vi "Main.vi"() -> ()   [LabVIEW 2019]
uses:
  <vilib>/vision/Image Controls.llb/IMAQ Image.ctl
  <vilib>/vision/NI_Vision_Development_Module.lvlib
panel:
  in  "Save Button":bool
  in  "Clear Button":bool
  in  "Image Path":path=path "D:/Krystian/Krystian/LabVIEW Data/OSP Projekt/Data/1.jpg" caption="Picture Path"
  in  "Exit":bool
  in  "Start":bool
  out "Results":string
  out "Image":T1(plugin-control)
  # "Application Panel"
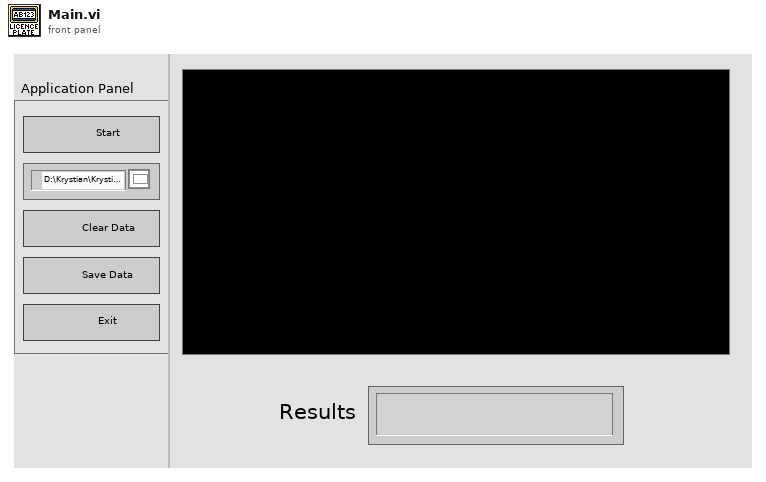
[diagram p1: front panel]
types:
  T1 = typedef "IMAQ Image.ctl" = refnum<image>
  T2 = enum32{"Invalid", "Standard", "Closed", "Hidden", "Minimized", "Maximized"}
  T3 = enum32{"invalid app kind", "Development System", "Run Time System", "Student Edition", "Embedded LabVIEW", "Evaluation", "Custom"}
  T4 = cluster{"Core":cluster{"Current VI Reference":refnum<vi>, "Close Panel on Exit?":bool}, "Your Boolean data":bool, "Results":string, "Image Path":path, "Data":cluster{"Rectangle":i32[]}, "Image":refnum<image>, "Python Path":path}
  T5 = cluster{"Current VI Reference":refnum<vi>, "Close Panel on Exit?":bool}
  T6 = typedef "Image Type" = u32
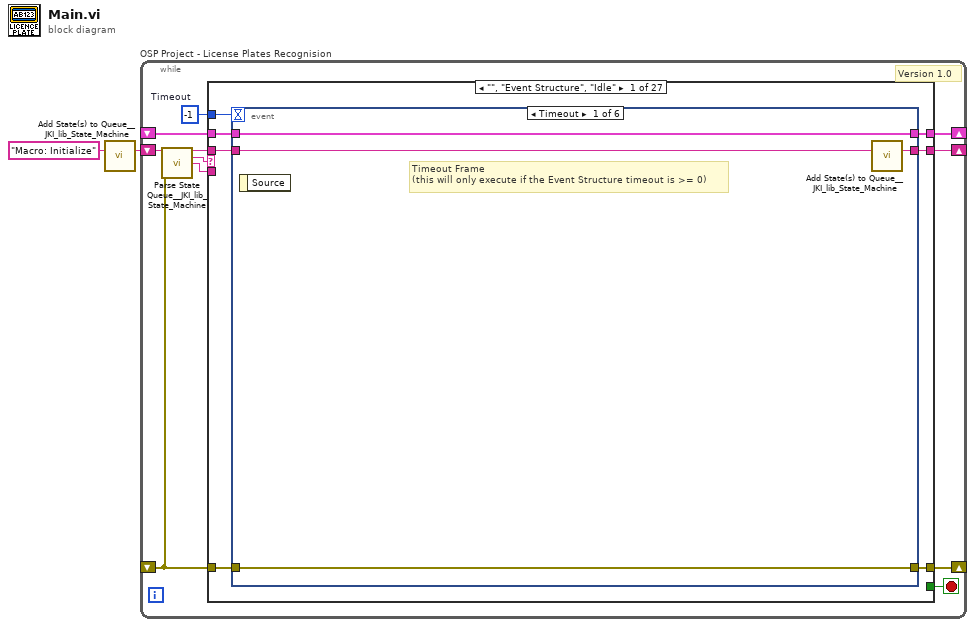
[diagram p0: block diagram]
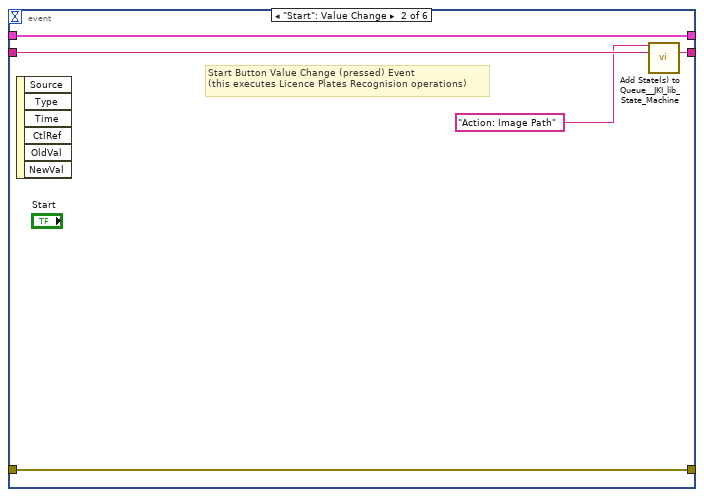
[diagram p2: hidden frame]
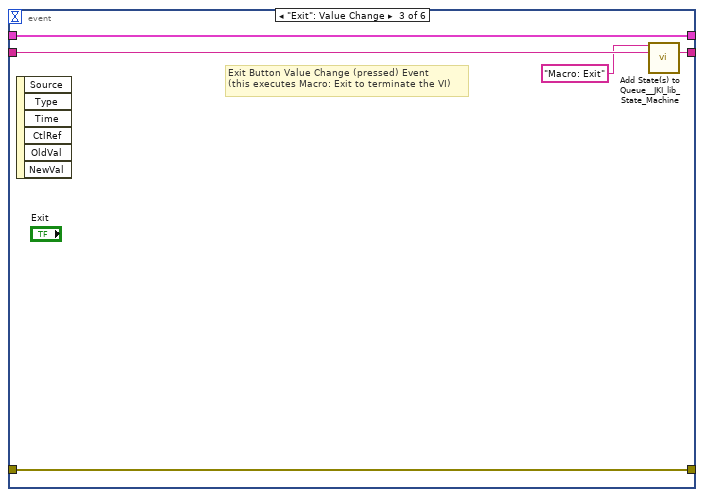
[diagram p3: hidden frame]
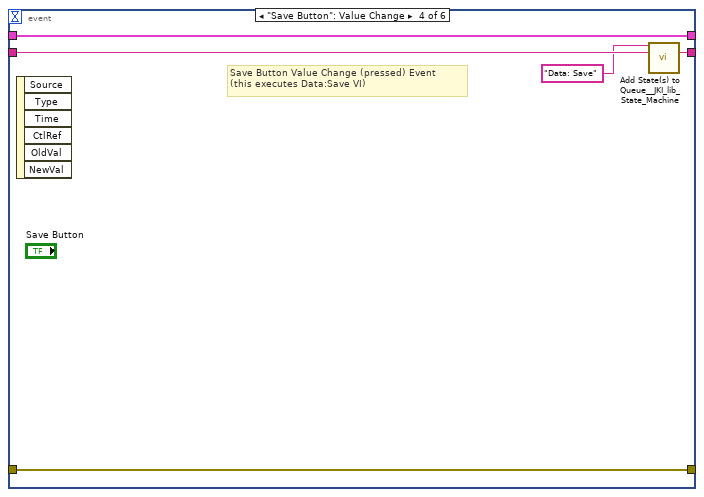
[diagram p4: hidden frame]
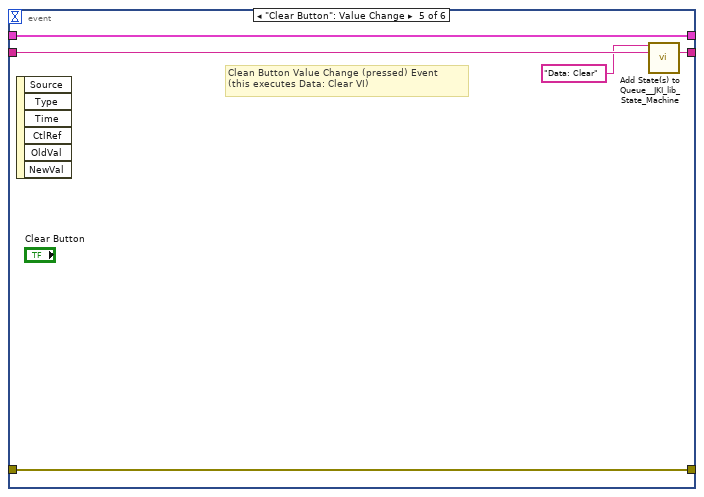
[diagram p5: hidden frame]
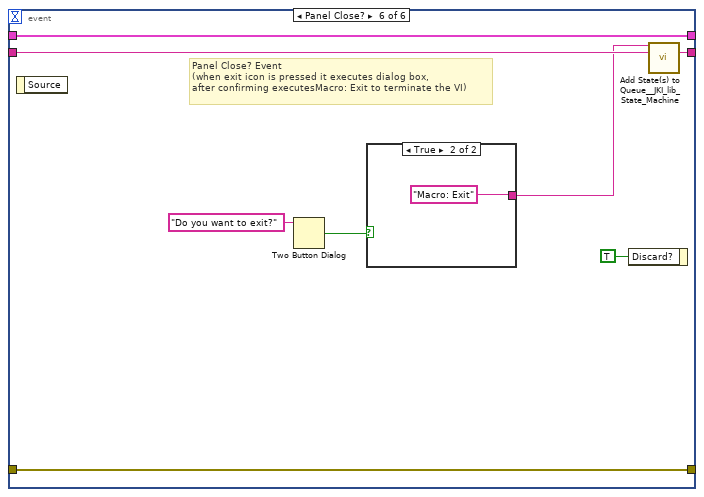
[diagram p6: hidden frame]
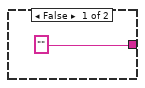
[diagram p7: hidden frame]
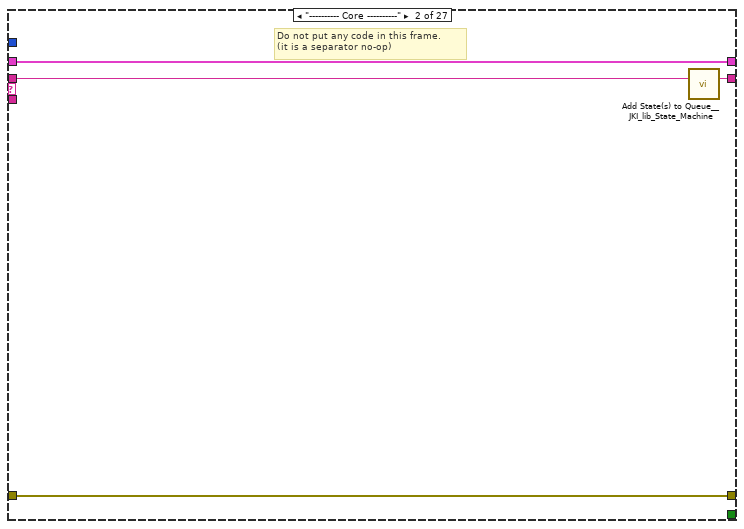
[diagram p8: hidden frame]
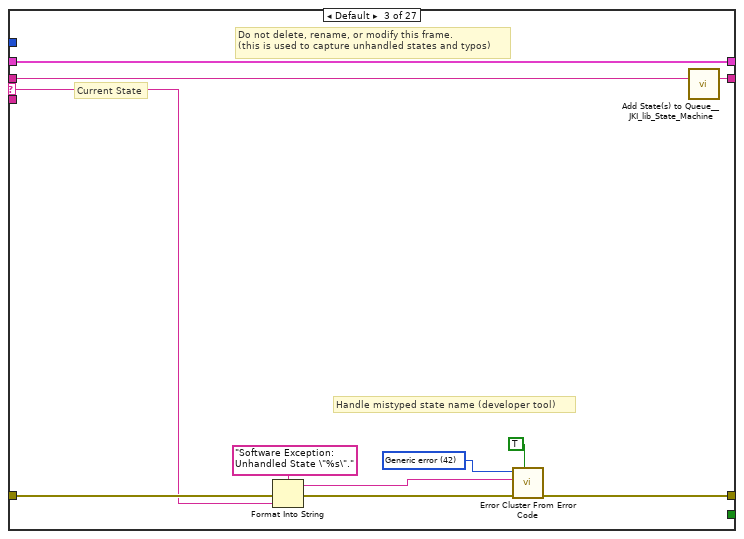
[diagram p9: hidden frame]
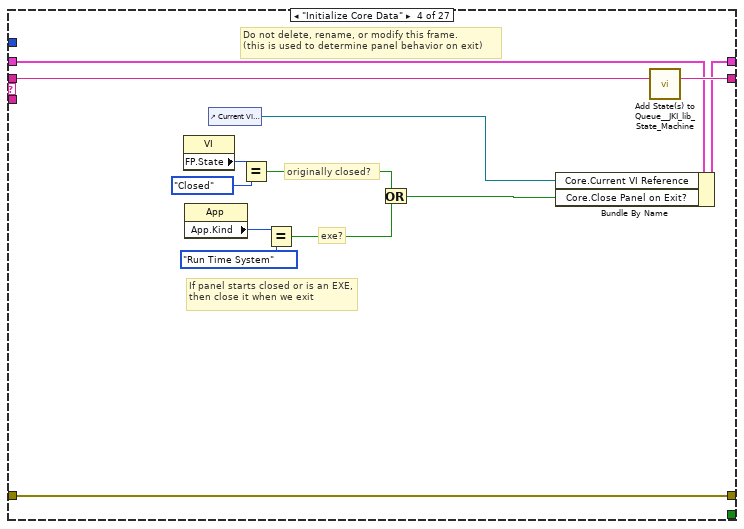
[diagram p10: hidden frame]
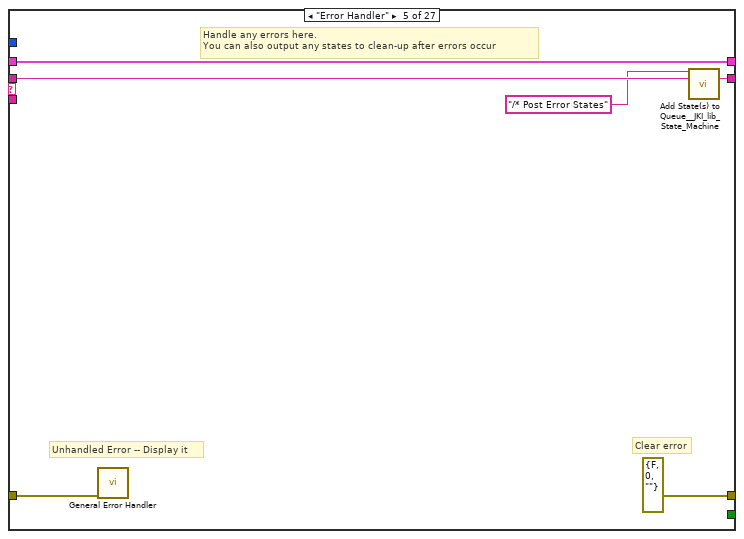
[diagram p11: hidden frame]
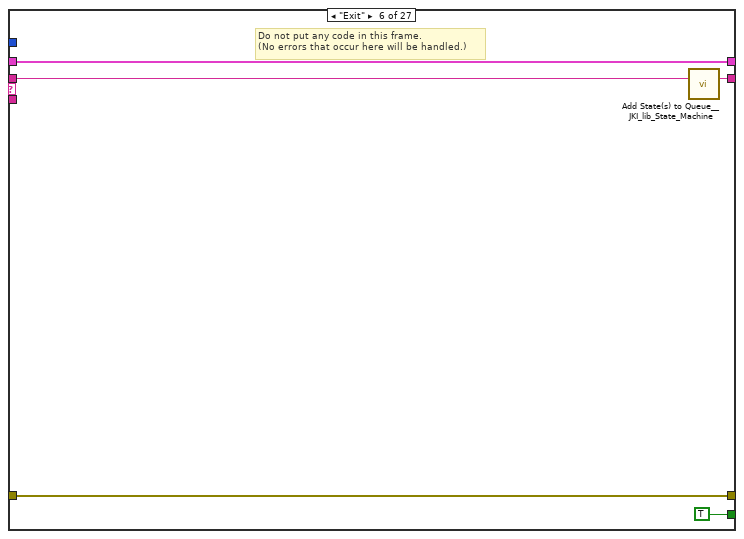
[diagram p12: hidden frame]
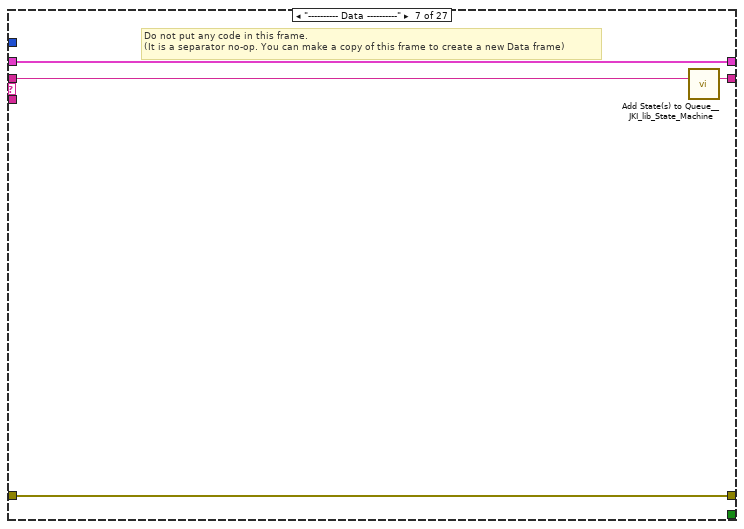
[diagram p13: hidden frame]
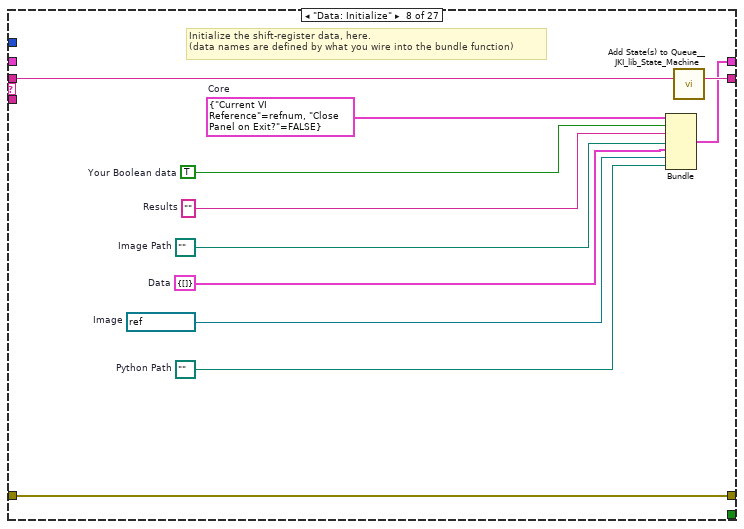
[diagram p14: hidden frame]
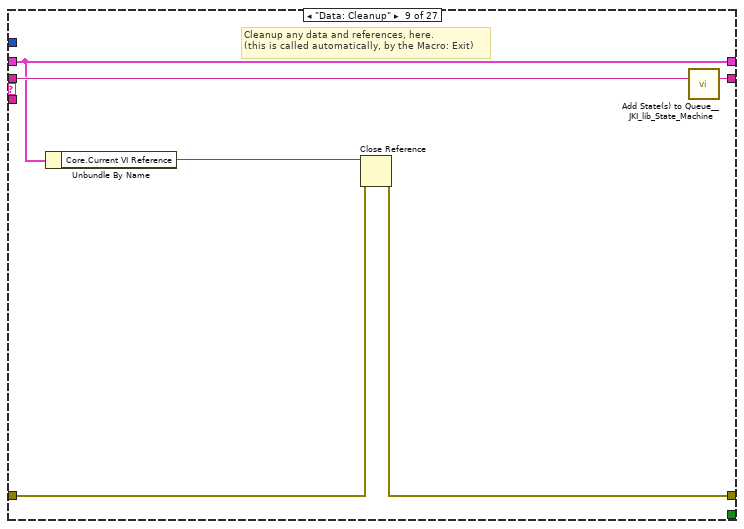
[diagram p15: hidden frame]
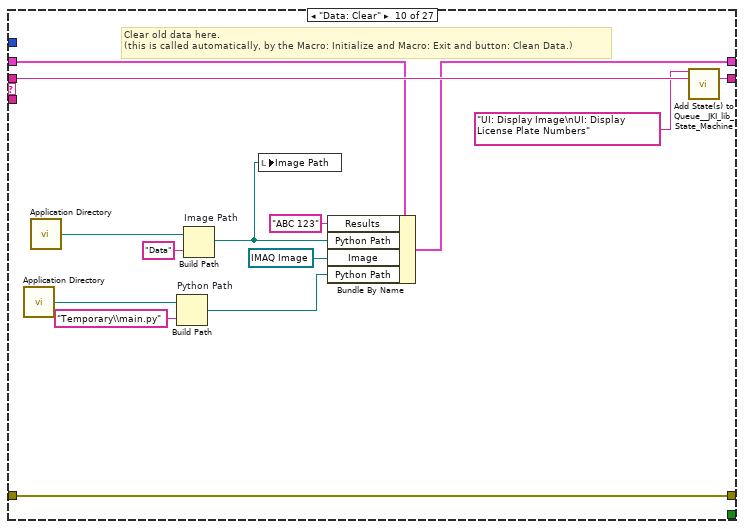
[diagram p16: hidden frame]
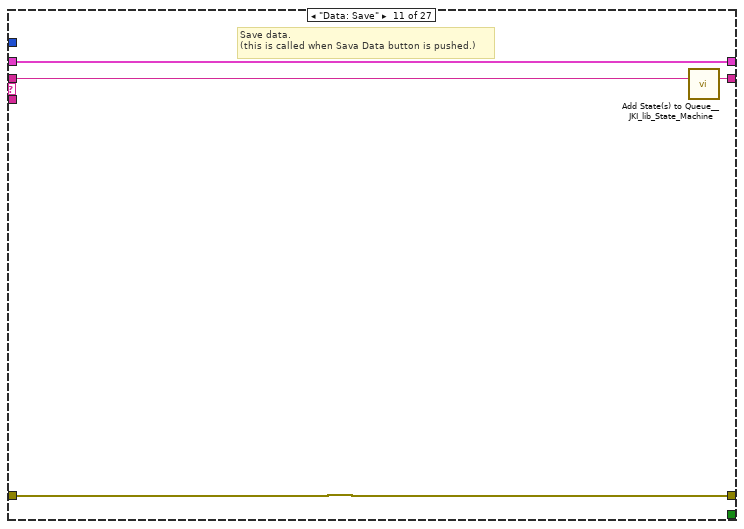
[diagram p17: hidden frame]
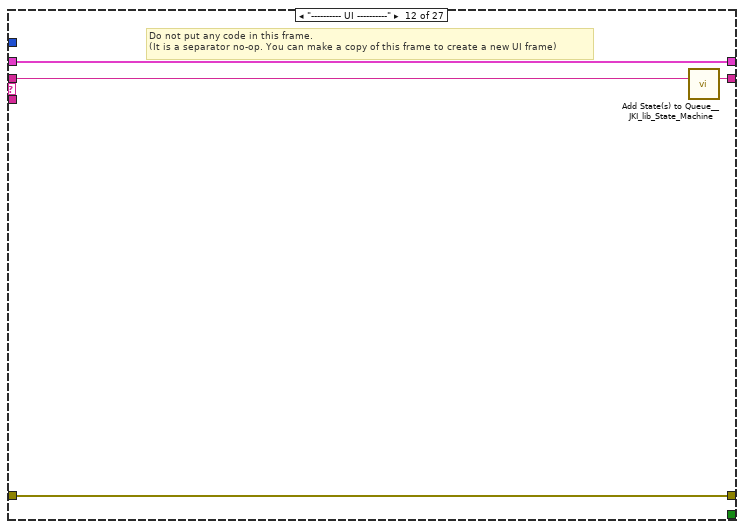
[diagram p18: hidden frame]
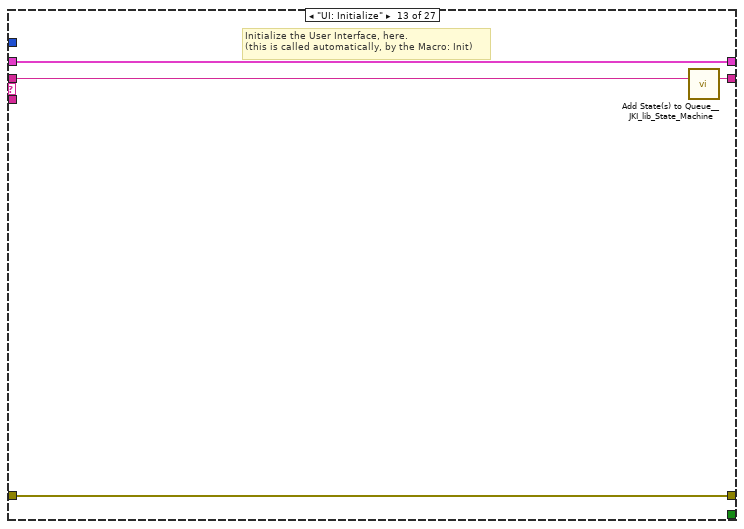
[diagram p19: hidden frame]
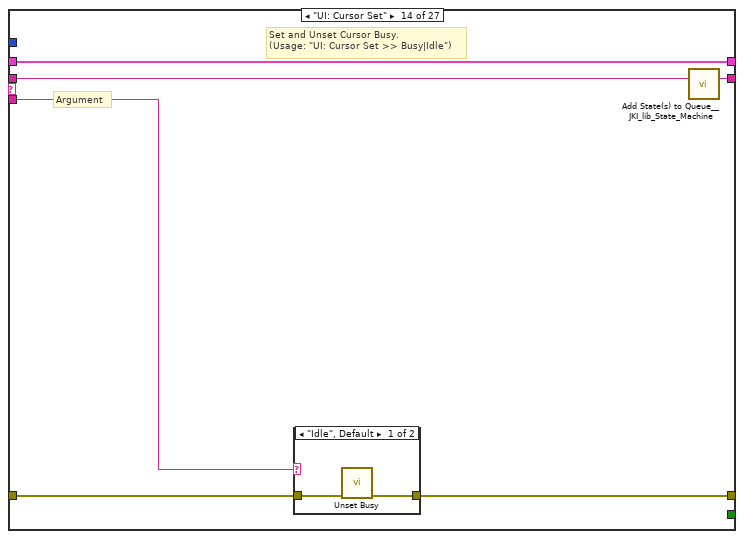
[diagram p20: hidden frame]
diagram:
  n1 = call <vilib>:"Add State(s) to Queue__JKI_lib_State_Machine.vi"("State(s) in (\"\")"="Macro: Initialize") -> ("States Out"=w2:string)  [unwired: 14 in]
  n2 = while "OSP Project - License Plates Recognision" {
    shift-right: [w6] -> _
    shift-left: _ -> [w5]
    shift-right: [w9] -> _
    shift-left: _ -> [w3]
    shift-right: [w8] -> _
    shift-left: w2 -> [w10]
    stop <- w7 stop-if-true
    w4 = -1  # Timeout
    # "Version 1.0"
    n3 = call <vilib>:"Parse State Queue__JKI_lib_State_Machine.vi"("State Queue"=w10, "Error In (no error)"=w3) -> ("Remaining States"=w12:string, "Current State"=w13:string, "Arguments"=w11:string)  [unwired: 11 in]
    n4 = case shown="\"\", \"Event Structure\", \"Idle\"" w13 {
      selector: w13 -> [_ _ w59 _ _ _ _ _ _ _ _ _ _ _ _ _ _ _ _ _ _ _ _ _ _ _ _]
      tunnel: w12 -> [w20 w58 w63 w82 w88 w93 w97 w108 w114 w128 w132 w136 w140 w146 w157 w227 w232 w236 w241 w251 w255 w265 w290 w299 w308 w319 w328]
      tunnel: w11 -> [_ _ _ _ _ _ _ _ _ _ _ _ _ w141 w151 _ _ _ _ _ _ _ _ _ _ _ _]
      tunnel: w5 -> [w18 w55 w61 w75 w85 w91 w94 _ w109 w124 w130 w133 w138 w144 w153 w224 w229 w233 w238 w248 w252 w261 w278 w293 w303 w311 w322]
      tunnel: [w17 w56 w65 w79 errorcluster {"status"=FALSE, "code"=0, "source"=""} ("error out") w90 w95 w105 w110 w126 w129 w134 w137 w142 w154 w225 w230 w234 w239 w249 w253 w263 w276 w297 w306 w317 w325] -> w9
      tunnel: w3 -> [w16 w56 w64 w79 w83 w90 w95 w105 w111 w126 w129 w134 w137 w143 w155 w225 w230 w234 w239 w249 w253 w263 w275 w297 w306 w317 w324]
      tunnel: [w19 w57 w62 w81 w87 w92 w96 w107 w113 w127 w131 w135 w139 w145 w156 w226 w231 w235 w240 w250 w254 w264 w289 w298 w307 w318 w327] -> w8
      tunnel: [_ _ _ _ _ TRUE _ _ _ _ _ _ _ _ _ _ _ _ _ _ _ _ _ _ _ _ _] -> w7
      tunnel: [w15 w55 w61 w80 w85 w91 w94 w106 w109 w125 w130 w133 w138 w144 w153 w224 w229 w233 w238 w248 w252 w262 w279 w294 w304 w312 w323] -> w6
      tunnel: w4 -> [w14 _ _ _ _ _ _ _ _ _ _ _ _ _ _ _ _ _ _ _ _ _ _ _ _ _ _]
      frame "", "Event Structure", "Idle" {
        n5 = event shown="[0] Timeout" {
          selector: _ -> [_ _ _ _ _ _]
          dyn-events: _ -> [_ _ _ _ _ _]
          timeout: w14 -> [_ _ _ _ _ _]
          tunnel: w20 -> [w24 w29 w34 w39 w44 w52]
          tunnel: [w23 w28 w33 w38 w43 w51] -> w19
          tunnel: w18 -> [w21 w26 w31 w36 w41 w49]
          tunnel: [w22 w27 w32 w37 w42 w50] -> w17
          tunnel: w16 -> [w22 w27 w32 w37 w42 w50]
          tunnel: [w21 w26 w31 w36 w41 w49] -> w15
          event Timeout {
            # "Timeout Frame\n(this will only execute if the Event Structure timeout is >= 0)"
            n6 = event-data() -> ()  [unwired: 1 in, 1 out]
            n7 = call <vilib>:"Add State(s) to Queue__JKI_lib_State_Machine.vi"("State(s) in (\"\")"=w24) -> ("States Out"=w23:string)  [unwired: 14 in]
          }
          event "Start": Value Change {
            # "Start Button Value Change (pressed) Event\n(this executes Licence Plates Recognision operations)"
            n8 = event-data() -> ()  [unwired: 1 in, 6 out]
            n9 = call <vilib>:"Add State(s) to Queue__JKI_lib_State_Machine.vi"("State(s) in Front (\"\")"="Action: Image Path", "State(s) in (\"\")"=w29) -> ("States Out"=w28:string)  [unwired: 13 in]
          }
          event "Exit": Value Change {
            # "Exit Button Value Change (pressed) Event\n(this executes Macro: Exit to terminate the VI)"
            n10 = event-data() -> ()  [unwired: 1 in, 6 out]
            n11 = call <vilib>:"Add State(s) to Queue__JKI_lib_State_Machine.vi"("State(s) in Front (\"\")"="Macro: Exit", "State(s) in (\"\")"=w34) -> ("States Out"=w33:string)  [unwired: 13 in]
          }
          event "Save Button": Value Change {
            # "Save Button Value Change (pressed) Event\n(this executes Data:Save VI)"
            n12 = event-data() -> ()  [unwired: 1 in, 6 out]
            n13 = call <vilib>:"Add State(s) to Queue__JKI_lib_State_Machine.vi"("State(s) in Front (\"\")"="Data: Save", "State(s) in (\"\")"=w39) -> ("States Out"=w38:string)  [unwired: 13 in]
          }
          event "Clear Button": Value Change {
            # "Clean Button Value Change (pressed) Event\n(this executes Data: Clear VI)"
            n14 = event-data() -> ()  [unwired: 1 in, 6 out]
            n15 = call <vilib>:"Add State(s) to Queue__JKI_lib_State_Machine.vi"("State(s) in Front (\"\")"="Data: Clear", "State(s) in (\"\")"=w44) -> ("States Out"=w43:string)  [unwired: 13 in]
          }
          event Panel Close? {
            # "Panel Close? Event\n(when exit icon is pressed it executes dialog box, \nafter confirming executesMacro: Exit to terminate the VI)"
            n16 = event-data() -> ()  [unwired: 1 in, 1 out]
            n17 = Two Button Dialog(message="Do you want to exit?") -> (T button?=w47:bool)  [unwired: 2 in]
            n18 = case shown="True" w47 {
              tunnel: ["" "Macro: Exit"] -> w45
              frame False {
              }
              frame True {
              }
            }
            n19 = event-data("Discard?"=TRUE) -> ()  [unwired: 1 in, 1 out]
            n20 = call <vilib>:"Add State(s) to Queue__JKI_lib_State_Machine.vi"("State(s) in Front (\"\")"=w45, "State(s) in (\"\")"=w52) -> ("States Out"=w51:string)  [unwired: 13 in]
          }
        }
      }
      frame "---------- Core ----------" {
        # "Do not put any code in this frame.\n(it is a separator no-op)"
        n21 = call <vilib>:"Add State(s) to Queue__JKI_lib_State_Machine.vi"("State(s) in (\"\")"=w58) -> ("States Out"=w57:string)  [unwired: 14 in]
      }
      frame Default {
        w68 = 42 items=["No error", "Argument error", "Memory is full", "Out of zone", "End of file", "File already open", "Generic file I/O error", "File not found", "File permission error", "Disk is full", "Duplicate path", "Too many files open", "System feature not enabled", "Resource file not found", "Cannot add resource", "Resource not found", "Image not found", "Image memory error", "Pen does not exist", "Config type invalid", "Config token not found", "Config parse error", "Config memory error", "Bad external code format", "Bad external code offset", "External code not present", "Null window", "Destroy window error", "Null menu", "Print aborted", "Bad print record", "Print driver error", "Windows error during printing", "Memory error during printing", "Print dialog error", "Generic print error", "Invalid device refnum", "Device not found", "Device parameter error", "Device unit error", "Cannot open device", "Device call aborted", "Generic error", "Cancelled by user", "Object ID too low", "Object ID too high", "Object not in heap", "Unknown heap", "Unknown object (invalid DefProc)", "Unknown object (DefProc not in table)", "Message out of range", "Invalid (null) method", "Unknown message", "Manager call not supported", "Bad address", "Network operation in progress", "Network operation timed out", "Connection is busy", "Network attribute not supported", "Network error", "Address in use", "System out of memory", "Connection aborted", "Connection refused", "Not connected", "Already connected", "Connection closed", "Initialization error (interapplication manager)", "Bad occurrence", "Wait on unbound occurrence handler", "Occurrence queue overflow", "Datalog type conflict", "Unused", "Unrecognized type (interapplication manager)", "Memory corrupt", "Failed to make temporary DLL", "Old CIN version", "Drag socket not found", "Failed to load drop-object", "Failed to register OLE object", "Failed to release OLE object", "Format specifier type mismatch", "Unknown format specifier", "Too few format specifiers", "Too many format specifiers", "Scan failed", "Newer CIN version", "Error converting to variant", "Runtime menu error", "Password tampered", "Variant attribute not found", "Incompatible variant data type", "Event data is not available", "Event Store is not present", "Occurrence is not found", "Event Queue is not created", "Event info is not available", "Refnum passed is NULL", "Error retrieving Class GUID", "Error retrieving CoClass GUID", "Error retrieving TypeLib GUID.", "Bad built application magic bytes.", "Specific driver is different from the specific driver associated with the Logical Name.", "There is no session opened to the class driver.", "Max Error", "MAX - Error with config objects", "MAX - Error loading configuration", "MAX - Group not supported"]
        # "Current State"
        # "Do not delete, rename, or modify this frame.\n(this is used to capture unhandled states and typos)"
        # "Handle mistyped state name (developer tool)"
        n22 = Format Into String(format string="Software Exception: Unhandled State \"%s\"." ("message"), error in=w64, w59) -> (resulting string=w67:string, error out=w66:errorcluster)  [unwired: 1 in]
        n23 = call <vilib>:"Error Cluster From Error Code.vi"("show call chain? (False)"=TRUE, "error in (no error)"=w66, "error message (\"\")"=w67, "error code (0)"=w68) -> ("error out"=w65:errorcluster)  [unwired: 5 in]
        n24 = call <vilib>:"Add State(s) to Queue__JKI_lib_State_Machine.vi"("State(s) in (\"\")"=w63) -> ("States Out"=w62:string)  [unwired: 14 in]
      }
      frame "Initialize Core Data" {
        # "Do not delete, rename, or modify this frame.\n(this is used to determine panel behavior on exit)"
        # "originally closed?"
        # "exe?"
        # "If panel starts closed or is an EXE, then close it when we exit"
        n25 = property class="VI"() -> ("FP.State"=w72:T2)  [unwired: 2 in, 2 out]
        n26 = property class="App"() -> ("App.Kind"=w78:T3)  [unwired: 2 in, 2 out]
        n27 = control-ref of="Current VI Reference"() -> (w73:refnum<vi>)
        n28 = Equal?(x=w72, y=T2."Closed" ("Front Panel Window:State")) -> (x = y?=w70:bool)
        n29 = Equal?(x=w78, y=T3."Run Time System" ("Application:Kind")) -> (x = y?=w76:bool)
        n30 = Or(x=w70, y=w76) -> (x .or. y?=w74:bool)
        n31 = Bundle By Name(cluster=w75, "Core.Current VI Reference"=w73, "Core.Close Panel on Exit?"=w74) -> (w80:T4)
        n32 = call <vilib>:"Add State(s) to Queue__JKI_lib_State_Machine.vi"("State(s) in (\"\")"=w82) -> ("States Out"=w81:string)  [unwired: 14 in]
      }
      frame "Error Handler" {
        # "Unhandled Error -- Display it"
        # "Handle any errors here.\nYou can also output any states to clean-up after errors occur"
        # "Clear error"
        n33 = call <vilib>:"General Error Handler.vi"("error in (no error)"=w83) -> ()  [unwired: 10 in, 5 out]
        n34 = call <vilib>:"Add State(s) to Queue__JKI_lib_State_Machine.vi"("State(s) in Front (\"\")"="/* Post Error States", "State(s) in (\"\")"=w88) -> ("States Out"=w87:string)  [unwired: 13 in]
      }
      frame "Exit" {
        # "Do not put any code in this frame.\n(No errors that occur here will be handled.)"
        n35 = call <vilib>:"Add State(s) to Queue__JKI_lib_State_Machine.vi"("State(s) in (\"\")"=w93) -> ("States Out"=w92:string)  [unwired: 14 in]
      }
      frame "---------- Data ----------" {
        # "Do not put any code in this frame.\n(It is a separator no-op. You can make a copy of this frame to create a new Data frame)"
        n36 = call <vilib>:"Add State(s) to Queue__JKI_lib_State_Machine.vi"("State(s) in (\"\")"=w97) -> ("States Out"=w96:string)  [unwired: 14 in]
      }
      frame "Data: Initialize" {
        w98 = path ""  # Python Path
        w99 = path ""  # Image Path
        w100 = refnum<image> refnum  # Image
        w101 = cluster{"Rectangle":i32[]} {"Rectangle"=[]}  # Data
        w102 = T5 {"Current VI Reference"=refnum, "Close Panel on Exit?"=FALSE}  # Core
        w104 = TRUE  # Your Boolean data
        w103 = ""  # Results
        # "Initialize the shift-register data, here.\n(data names are defined by what you wire into the bundle function)"
        n37 = Bundle("Core"=w102, "Your Boolean data"=w104, "Results"=w103, "Image Path"=w99, "Data"=w101, "Image"=w100, "Python Path"=w98) -> (w106:T4)  [unwired: 1 in]
        n38 = call <vilib>:"Add State(s) to Queue__JKI_lib_State_Machine.vi"("State(s) in (\"\")"=w108) -> ("States Out"=w107:string)  [unwired: 14 in]
      }
      frame "Data: Cleanup" {
        # "Cleanup any data and references, here.\n(this is called automatically, by the Macro: Exit)"
        n39 = Unbundle By Name(w109) -> ("Core.Current VI Reference"=w112:refnum<vi>)
        n40 = Close Reference(reference=w112, error in (no error)=w111) -> (error out=w110:errorcluster)
        n41 = call <vilib>:"Add State(s) to Queue__JKI_lib_State_Machine.vi"("State(s) in (\"\")"=w114) -> ("States Out"=w113:string)  [unwired: 14 in]
      }
      frame "Data: Clear" {
        # "Clear old data here.\n(this is called automatically, by the Macro: Initialize and Macro: Exit and button: Clean Data.)"
        n42 = call <vilib>:"Application Directory.vi"() -> ("Application Directory"=w117:path)
        n43 = call <vilib>:"Application Directory.vi"() -> ("Application Directory"=w120:path)
        n44 = Build Path "Python Path"(base path=w117, name or relative path="Temporary\\main.py") -> (appended path=w115:path)
        n45 = Build Path "Image Path"(base path=w120, name or relative path="Data") -> (appended path=w118:path)
        n46 = local write "Image Path"(w118) -> ()
        n47 = Bundle By Name(cluster=w124, "Results"="ABC 123", "Python Path"=w118, "Image"=T1 refnum, "Python Path"=w115) -> (w125:T4)
        n48 = call <vilib>:"Add State(s) to Queue__JKI_lib_State_Machine.vi"("State(s) in Front (\"\")"="UI: Display Image\nUI: Display License Plate Numbers", "State(s) in (\"\")"=w128) -> ("States Out"=w127:string)  [unwired: 13 in]
      }
      frame "Data: Save" {
        # "Save data.\n(this is called when Sava Data button is pushed.)"
        n49 = call <vilib>:"Add State(s) to Queue__JKI_lib_State_Machine.vi"("State(s) in (\"\")"=w132) -> ("States Out"=w131:string)  [unwired: 14 in]
      }
      frame "---------- UI ----------" {
        # "Do not put any code in this frame.\n(It is a separator no-op. You can make a copy of this frame to create a new UI frame)"
        n50 = call <vilib>:"Add State(s) to Queue__JKI_lib_State_Machine.vi"("State(s) in (\"\")"=w136) -> ("States Out"=w135:string)  [unwired: 14 in]
      }
      frame "UI: Initialize" {
        # "Initialize the User Interface, here.\n(this is called automatically, by the Macro: Init)"
        n51 = call <vilib>:"Add State(s) to Queue__JKI_lib_State_Machine.vi"("State(s) in (\"\")"=w140) -> ("States Out"=w139:string)  [unwired: 14 in]
      }
      frame "UI: Cursor Set" {
        # "Argument"
        # "Set and Unset Cursor Busy.\n(Usage: \"UI: Cursor Set >> Busy|Idle\")"
        n52 = case shown="\"Idle\", Default" w141 {
          tunnel: w143 -> [w148 w150]
          tunnel: [w147 w149] -> w142
          frame "Idle", Default {
            n53 = call <vilib>:"Unset Busy.vi"("error in (no error)"=w148) -> ("error out"=w147:errorcluster)  [unwired: 10 in]
          }
          frame "Busy" {
            n54 = call <vilib>:"Set Busy.vi"("error in (no error)"=w150) -> ("error out"=w149:errorcluster)  [unwired: 9 in, 1 out]
          }
        }
        n55 = call <vilib>:"Add State(s) to Queue__JKI_lib_State_Machine.vi"("State(s) in (\"\")"=w146) -> ("States Out"=w145:string)  [unwired: 14 in]
      }
      frame "UI: Front Panel State" {
        # "Argument"
        # "Set Front Panel Open or Closed\n(Usage: \"UI: Front Panel State >> Open|Close\")"
        n56 = Unbundle By Name(w153) -> ("Core.Current VI Reference"=w152:refnum<vi>)
        n57 = case shown="\"Minimize\", \"Minimized\"" w151 {
          tunnel: w155 -> [w163 w178 w189 w202 w215]
          tunnel: [w165 w179 w191 w204 w217] -> w154
          tunnel: w152 -> [w164 w176 w190 w203 w216]
          frame "Open", "Standard", Default {
            w158 = T2."Standard" ("State")
            n58 = property class="VI"(reference=w164, error in=w163) -> (reference out=w161:refnum<vi>, error out=w162:errorcluster, "FP.State"=w160:T2)
            n59 = Not Equal?(x=w160, y=w158) -> (x != y?=w159:bool)
            n60 = case shown="True" w159 {
              tunnel: [w169 w171] -> w165
              tunnel: w162 -> [w168 w171]
              tunnel: w161 -> [w167 _]
              tunnel: w158 -> [w166 _]
              frame True {
                n61 = invoke class="VI" method="FP.Open"(reference=w167, error in=w168, "Activate"=TRUE, "State"=w166) -> (error out=w169:errorcluster)  [unwired: 1 in, 4 out]
              }
              frame False {
              }
            }
          }
          frame "Close", "Closed" {
            n62 = property class="VI"(reference=w176, error in=w178) -> (reference out=w175:refnum<vi>, error out=w177:errorcluster, "FP.State"=w173:T2)
            n63 = Not Equal?(x=w173, y=T2."Closed" ("Front Panel Window:State")) -> (x != y?=w172:bool)
            n64 = case shown="True" w172 {
              tunnel: [w180 w183] -> w179
              tunnel: w177 -> [w180 w182]
              tunnel: w175 -> [_ w181]
              frame False {
              }
              frame True {
                n65 = invoke class="VI" method="FP.Close"(reference=w181, error in=w182) -> (error out=w183:errorcluster)  [unwired: 1 in, 2 out]
              }
            }
          }
          frame "Hidden", "Hide" {
            w184 = T2."Hidden" ("State")
            n66 = property class="VI"(reference=w190, error in=w189) -> (reference out=w187:refnum<vi>, error out=w188:errorcluster, "FP.State"=w186:T2)
            n67 = Not Equal?(x=w186, y=w184) -> (x != y?=w185:bool)
            n68 = case shown="True" w185 {
              tunnel: [w195 w196] -> w191
              tunnel: w188 -> [w194 w196]
              tunnel: w187 -> [w193 _]
              tunnel: w184 -> [w192 _]
              frame True {
                n69 = invoke class="VI" method="FP.Open"(reference=w193, error in=w194, "State"=w192) -> (error out=w195:errorcluster)  [unwired: 2 in, 4 out]
              }
              frame False {
              }
            }
          }
          frame "Minimize", "Minimized" {
            w197 = T2."Minimized" ("State")
            n70 = property class="VI"(reference=w203, error in=w202) -> (reference out=w200:refnum<vi>, error out=w201:errorcluster, "FP.State"=w199:T2)
            n71 = Not Equal?(x=w199, y=w197) -> (x != y?=w198:bool)
            n72 = case shown="True" w198 {
              tunnel: [w208 w209] -> w204
              tunnel: w201 -> [w207 w209]
              tunnel: w200 -> [w206 _]
              tunnel: w197 -> [w205 _]
              frame True {
                n73 = invoke class="VI" method="FP.Open"(reference=w206, error in=w207, "State"=w205) -> (error out=w208:errorcluster)  [unwired: 2 in, 4 out]
              }
              frame False {
              }
            }
          }
          frame "Maximize", "Maximized" {
            w210 = T2."Maximized" ("State")
            n74 = property class="VI"(reference=w216, error in=w215) -> (reference out=w213:refnum<vi>, error out=w214:errorcluster, "FP.State"=w212:T2)
            n75 = Not Equal?(x=w212, y=w210) -> (x != y?=w211:bool)
            n76 = case shown="True" w211 {
              tunnel: [w221 w222] -> w217
              tunnel: w214 -> [w220 w222]
              tunnel: w213 -> [w219 _]
              tunnel: w210 -> [w218 _]
              frame True {
                n77 = invoke class="VI" method="FP.Open"(reference=w219, error in=w220, "State"=w218) -> (error out=w221:errorcluster)  [unwired: 2 in, 4 out]
              }
              frame False {
              }
            }
          }
        }
        n78 = call <vilib>:"Add State(s) to Queue__JKI_lib_State_Machine.vi"("State(s) in (\"\")"=w157) -> ("States Out"=w156:string)  [unwired: 14 in]
      }
      frame "UI: Display Image" {
        # "Display Image\n(In this frame Image is displayed on UI.)"
        n79 = Unbundle By Name(w224) -> ("Image"=→"Image":refnum<image>)
        n80 = call <vilib>:"Add State(s) to Queue__JKI_lib_State_Machine.vi"("State(s) in (\"\")"=w227) -> ("States Out"=w226:string)  [unwired: 14 in]
      }
      frame "UI: Display License Plate Numbers" {
        # "Display License Plate Numbers\n(In this frame Resoults are displayed on UI.)"
        n81 = Unbundle By Name(w229) -> ("Results"=→"Results":string)
        n82 = call <vilib>:"Add State(s) to Queue__JKI_lib_State_Machine.vi"("State(s) in (\"\")"=w232) -> ("States Out"=w231:string)  [unwired: 14 in]
      }
      frame "---------- Macro ----------" {
        # "Do not put any code in this frame.\n(It is a separator no-op. You can make a copy of this frame to create a new Macro frame)"
        n83 = call <vilib>:"Add State(s) to Queue__JKI_lib_State_Machine.vi"("State(s) in (\"\")"=w236) -> ("States Out"=w235:string)  [unwired: 14 in]
      }
      frame "Macro: Initialize" {
        w237 = "Data: Initialize\nInitialize Core Data\nData: Clear\nUI: Initialize\nUI: Front Panel State >> Open"  # Data: Initialize Initialize Core Data Data: Clear UI: Initialize UI: Front Panel State >> Open
        # "Initialization Macro\n(This is called once, when the VI starts)"
        n84 = call <vilib>:"Add State(s) to Queue__JKI_lib_State_Machine.vi"("State(s) in Front (\"\")"=w237, "State(s) in (\"\")"=w241) -> ("States Out"=w240:string)  [unwired: 13 in]
      }
      frame "Macro: Exit" {
        # "Exit Macro\n(This is called once, when the VI exits)"
        n85 = Unbundle By Name(w248) -> ("Core.Close Panel on Exit?"=w247:bool)
        n86 = Select(t="UI: Front Panel State >> Close", s=w247, f="") -> (s? t:f=w244:string)
        n87 = call <vilib>:"Add State(s) to Queue__JKI_lib_State_Machine.vi"("State(s) in (\"\")"=w244, "State(s) at Back (\"\")"="Data: Cleanup\nData: Clear\nExit") -> ("States Out"=w242:string)  [unwired: 13 in]
        n88 = call <vilib>:"Add State(s) to Queue__JKI_lib_State_Machine.vi"("State(s) in Front (\"\")"=w242, "State(s) in (\"\")"=w251) -> ("States Out"=w250:string)  [unwired: 13 in]
      }
      frame "---------- Action ----------" {
        # "Template Separator\n(You can make a copy of, or modify, this frame)"
        n89 = call <vilib>:"Add State(s) to Queue__JKI_lib_State_Machine.vi"("State(s) in (\"\")"=w255) -> ("States Out"=w254:string)  [unwired: 14 in]
      }
      frame "Action: Image Path" {
        w260 = path ""  # Empty Path Constant
        # "Image Path.\n(Checking if Image Path is correct.)"
        n90 = Equal?(x="Image Path", y=w260) -> (x = y?=w259:bool)
        n91 = case shown="True" w259 {
          tunnel: "Image Path" -> [w268 _]
          tunnel: [w269 TRUE] -> w256
          frame False {
            w270 = "jpg" ("search string/char (-)")
            n92 = Path To String(path=w268) -> (string=w271:string)
            n93 = Search/Split String(string=w271, search string/char (-)=w270) -> (match + rest of string=w272:string)  [unwired: 1 in, 2 out]
            n94 = Equal?(x=w272, y=w270) -> (x = y?=w269:bool)
          }
          frame True {
            n95 = One Button Dialog(message="Image path is EMPTY!\nPlease select image path.") -> ()  [unwired: 1 in, 1 out]
          }
        }
        n96 = Bundle By Name(cluster=w261, "Image Path"="Image Path") -> (w262:T4)
        n97 = case shown="False" w256 {
          tunnel: [_ "Action: Python Code"] -> w257
          frame False {
            n98 = One Button Dialog(message="Image path is NOT CORRECT!\nPlease select JPG image.") -> ()  [unwired: 1 in, 1 out]
          }
          frame True {
          }
        }
        n99 = call <vilib>:"Add State(s) to Queue__JKI_lib_State_Machine.vi"("State(s) in Front (\"\")"=w257, "State(s) in (\"\")"=w265) -> ("States Out"=w264:string)  [unwired: 13 in]
      }
      frame "Action: Python Code" {
        w285 = "find_plate"  # function name
        w288 = "3.6"  # Python version
        # "Python Code.\n(In this frame we are using Python Node to identify coordinates of license plate.)"
        n100 = Unbundle By Name(w278) -> ("Image Path"=w281:path)
        n101 = Unbundle By Name(w278) -> ("Data.Rectangle"=w283:i32[])
        n102 = Unbundle By Name(w278) -> ("Python Path"=w282:path)
        n103 = Open Python Session(python version=w288) -> (session out=w287:refnum<k35>)  [unwired: 2 in, 1 out]
        n104 = Path To String(path=w281) -> (string=w284:string)
        n105 = node(w287, w282, w285, w275, w283, w284) -> (w286:refnum<k35>, w276:errorcluster, w280:i32[])  [unwired: 1 in, 2 out]
        n106 = Close Python Session(session in=w286) -> ()  [unwired: 1 in, 1 out]
        n107 = Bundle By Name(cluster=w278, "Data.Rectangle"=w280) -> (w279:T4)
        n108 = call <vilib>:"Add State(s) to Queue__JKI_lib_State_Machine.vi"("State(s) in Front (\"\")"="Action: IMAQ Create" ("State(s) in Front (\"\")"), "State(s) in (\"\")"=w290) -> ("States Out"=w289:string)  [unwired: 13 in]
      }
      frame "Action: IMAQ Create" {
        w295 = T6 4 items=["Grayscale (U8)", "Grayscale (I16)", "Grayscale (SGL)", "Complex (CSG)", "RGB (U32)", "HSL (U32)", "RGB (U64)", "Grayscale (U16)"] ("Image Type")
        w296 = "untitled"  # Image Name
        # "IMAQ Create.\n(In this frame it is created a temorary memory location for an image.)"
        n109 = call "IMAQ Create"("Image Name"=w296, "Image Type"=w295) -> ("New Image"=w292:T1)  [unwired: 3 in, 1 out]
        n110 = Bundle By Name(cluster=w293, "Image"=w292) -> (w294:T4)
        n111 = call <vilib>:"Add State(s) to Queue__JKI_lib_State_Machine.vi"("State(s) in Front (\"\")"="Action: IMAQ Read FIle" ("State(s) in Front (\"\")"), "State(s) in (\"\")"=w299) -> ("States Out"=w298:string)  [unwired: 13 in]
      }
      frame "Action: IMAQ Read FIle" {
        # "IMAQ Read File.\n(In this frame image file is being read.)"
        n112 = Unbundle By Name(w303) -> ("Image"=w302:refnum<image>)
        n113 = Unbundle By Name(w303) -> ("Image Path"=w305:path)
        n114 = call "IMAQ ReadFile 2.vi"("File Path"=w305, "Image"=w302) -> ("Image Out"=w300:T1)  [unwired: 5 in, 4 out]
        n115 = Bundle By Name(cluster=w303, "Image"=w300) -> (w304:T4)
        n116 = call <vilib>:"Add State(s) to Queue__JKI_lib_State_Machine.vi"("State(s) in Front (\"\")"="Action: IMAQ Extract" ("State(s) in Front (\"\")"), "State(s) in (\"\")"=w308) -> ("States Out"=w307:string)  [unwired: 13 in]
      }
      frame "Action: IMAQ Extract" {
        w309 = 1  # Y Step Size
        w315 = 1  # X Step Size
        # "IMAQ Extract.\n(In this frame part of image is extracted with adjustment of the horizontal and vertical resolution.)"
        n117 = Unbundle By Name(w311) -> ("Data.Rectangle"=w314:i32[])
        n118 = Unbundle By Name(w311) -> ("Image"=w316:refnum<image>)
        n119 = call "IMAQ Extract 2"("Y Step Size"=w309, "Optional Rectangle"=w314, "X Step Size"=w315, "Image Src"=w316) -> ("Image Dst Out"=w313:T1)  [unwired: 6 in, 1 out]
        n120 = Bundle By Name(cluster=w311, "Image"=w313) -> (w312:T4)
        n121 = call <vilib>:"Add State(s) to Queue__JKI_lib_State_Machine.vi"("State(s) in Front (\"\")"="UI: Display Image\nAction: IMAQ OCR", "State(s) in (\"\")"=w319) -> ("States Out"=w318:string)  [unwired: 13 in]
      }
      frame "Action: IMAQ OCR" {
        # "IMAQ OCR.\n(In this frame the optical character recognition is being used.)"
        n122 = Unbundle By Name(w322) -> ("Image"=w326:refnum<image>)
        n123 = call "IMAQ OCR.vi"("Image In"=w326, "error in"=w324) -> ("String (OCR/OCV 2)"=w321:string, "error out"=w325:errorcluster)  [unwired: 24 in]
        n124 = Bundle By Name(cluster=w322, "Results"=w321) -> (w323:T4)
        n125 = call <vilib>:"Add State(s) to Queue__JKI_lib_State_Machine.vi"("State(s) in Front (\"\")"="UI: Display License Plate Numbers" ("State(s) in Front (\"\")"), "State(s) in (\"\")"=w328) -> ("States Out"=w327:string)  [unwired: 13 in]
      }
    }
  }
